vi "Unsigned Unsafe Subtract.vi"(1 "B":T1={"Array Num"=[1, 2, 3], "Decimal Index"=0, "stop"=FALSE}, 2 "A":T1={"Array Num"=[1, 2, 3], "Decimal Index"=0, "stop"=FALSE}) -> (0 "A-B":T1={"Array Num"=[1, 2, 3], "Decimal Index"=0, "stop"=FALSE})   [LabVIEW 2025]
uses:
  Number.ctl
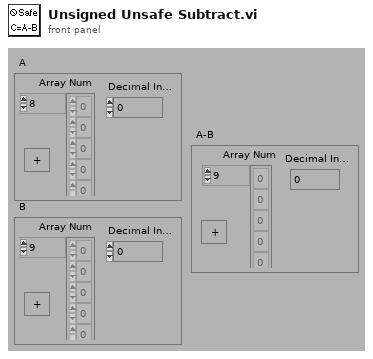
[diagram p1: front panel]
types:
  T1 = typedef "Number.ctl" = cluster{"Array Num":i8[], "Decimal Index":i32, "stop":bool}
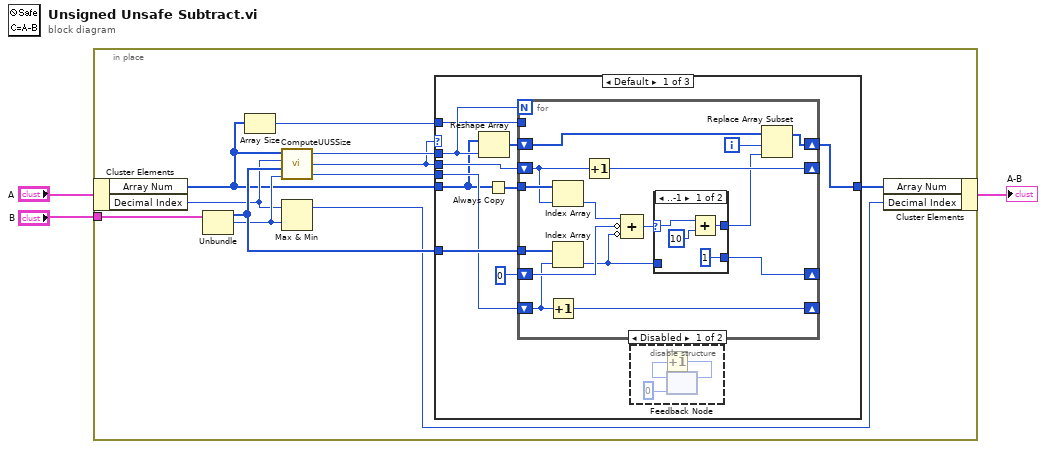
[diagram p0: block diagram]
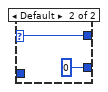
[diagram p3: hidden frame]
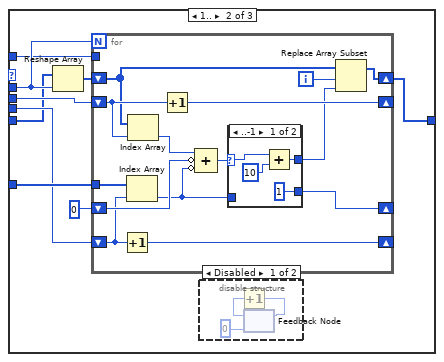
[diagram p4: hidden frame]
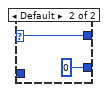
[diagram p6: hidden frame]
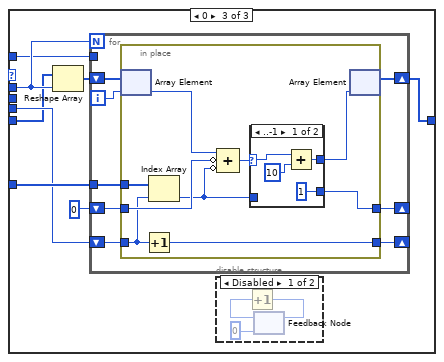
[diagram p7: hidden frame]
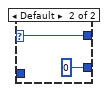
[diagram p9: hidden frame]
diagram:
  n1 = in-place {
    in-place-border: "B" -> [w14]
    n2 = in-place-cluster #1("A") -> ("Array Num"=w6:i8[], "Decimal Index"=w10:i32)
    n3 = Unbundle(w14) -> ("Array Num"=w13:i8[], "Decimal Index"=w12:i32)  [unwired: 1 out]
    n4 = Array Size(array=w6) -> (size(s)=w5:i32)
    n5 = call "ComputeUUSSize.vi"("B Array Position"=w12, "BArray"=w13, "A Array Position"=w10, "A Array Num"=w6) -> ("B Index"=w11:i32, "A Index"=w4:i32, "Loop Count"=w8:i32)
    n6 = Max & Min(x=w10, y=w12) -> (max(x,y)=w9:i32)  [unwired: 1 out]
    n7 = case shown="Default" w4 {
      tunnel: w13 -> [w23 w56 w87]
      tunnel: w4 -> [w22 w55 _]
      tunnel: w11 -> [w21 w54 w86]
      tunnel: w8 -> [w19 w53 w85]
      tunnel: [w17 w51 w83] -> w7
      tunnel: w6 -> [w16 w50 w81]
      tunnel: w5 -> [w15 w49 w82]
      frame Default {
        n8 = Reshape Array(w16, w19) -> (w18:i8[])
        n9 = Always Copy(1:w16) -> (0:w20:i8[])
        n10 = for {
          N: w19 -> [_]
          tunnel: w23 -> [w42]
          shift-right: [w41] -> _
          shift-left: i8 0 -> [w35]
          tunnel: w20 -> [w40]
          shift-right: [w37] -> _
          shift-left: w22 -> [w39]
          shift-right: [w38] -> _
          shift-left: w21 -> [w32]
          shift-right: [w30] -> w17
          shift-left: w18 -> [w31]
          tunnel: w15 -> [_]
          i -> [w29]
          n11 = Increment(x=w32) -> (x+1=w38:i32)
          n12 = Index Array(array=w40, index=w39) -> (element=w36:i8)
          n13 = Index Array(array=w42, index=w32) -> (element=w34:i8)
          n14 = Increment(x=w39) -> (x+1=w37:i32)
          n15 = Compound Arithmetic op=ADD(w36, invert w35, invert w34) -> (w33:i8)
          n16 = case shown="..-1" w33 {
            selector: w33 -> [w43 w47]
            tunnel: w34 -> [_ _]
            tunnel: [i8 1 i8 0] -> w41
            tunnel: [w44 w47] -> w28
            frame ..-1 {
              n17 = Add(x=w43, y=i8 10) -> (x+y=w44:i8)
            }
            frame Default {
            }
          }
          n18 = Replace Array Subset(array=w31, new element=w28, index=w29) -> (w30:i8[])
        }
        n19 = disable-structure shown="Disabled" {
          frame Disabled {
            n20 = feedback #2(0) -> (w26:i32)
            n21 = Increment(x=w26) -> (x+1=w27:i32)
            n22 = feedback-in #2(w27) -> ()
          }
          frame Enabled {
          }
        }
      }
      frame 1.. {
        n23 = Reshape Array(w50, w53) -> (w52:i8[])
        n24 = for {
          N: w53 -> [_]
          tunnel: w56 -> [w74]
          shift-right: [w73] -> _
          shift-left: i8 0 -> [w68]
          shift-right: [w70] -> _
          shift-left: w55 -> [w72]
          shift-right: [w71] -> _
          shift-left: w54 -> [w65]
          shift-right: [w64] -> w51
          shift-left: w52 -> [w61]
          tunnel: w49 -> [_]
          i -> [w63]
          n25 = Increment(x=w65) -> (x+1=w71:i32)
          n26 = Index Array(array=w74, index=w65) -> (element=w67:i8)
          n27 = Index Array(array=w61, index=w72) -> (element=w69:i8)
          n28 = Increment(x=w72) -> (x+1=w70:i32)
          n29 = Compound Arithmetic op=ADD(w69, invert w68, invert w67) -> (w66:i8)
          n30 = case shown="..-1" w66 {
            selector: w66 -> [w75 w79]
            tunnel: w67 -> [_ _]
            tunnel: [i8 1 i8 0] -> w73
            tunnel: [w76 w79] -> w62
            frame ..-1 {
              n31 = Add(x=w75, y=i8 10) -> (x+y=w76:i8)
            }
            frame Default {
            }
          }
          n32 = Replace Array Subset(array=w61, new element=w62, index=w63) -> (w64:i8[])
        }
        n33 = disable-structure shown="Disabled" {
          frame Disabled {
            n34 = feedback #3(0) -> (w58:i32)
            n35 = Increment(x=w58) -> (x+1=w59:i32)
            n36 = feedback-in #3(w59) -> ()
          }
          frame Enabled {
          }
        }
      }
      frame 0 {
        n37 = Reshape Array(w81, w85) -> (w84:i8[])
        n38 = for {
          N: w85 -> [_]
          tunnel: w87 -> [w99]
          shift-right: [w98] -> _
          shift-left: i8 0 -> [w96]
          shift-right: [w97] -> _
          shift-left: w86 -> [w95]
          shift-right: [w92] -> w83
          shift-left: w84 -> [w94]
          tunnel: w82 -> [_]
          i -> [w93]
          n39 = in-place {
            in-place-border: w99 -> [w108]
            in-place-border: [w107] -> w98
            in-place-border: [w106] -> w97
            in-place-border: w96 -> [w105]
            in-place-border: w95 -> [w102]
            n40 = in-place-array #4(w94, w93) -> (w100:i8)
            n41 = Increment(x=w102) -> (x+1=w106:i32)
            n42 = Index Array(array=w108, index=w102) -> (element=w104:i8)
            n43 = Compound Arithmetic op=ADD(w100, invert w105, invert w104) -> (w103:i8)
            n44 = case shown="..-1" w103 {
              selector: w103 -> [w109 w113]
              tunnel: w104 -> [_ _]
              tunnel: [i8 1 i8 0] -> w107
              tunnel: [w110 w113] -> w101
              frame ..-1 {
                n45 = Add(x=w109, y=i8 10) -> (x+y=w110:i8)
              }
              frame Default {
              }
            }
            n46 = in-place-array #4(w101) -> (w92:i8[])  [unwired: 1 out]
          }
        }
        n47 = disable-structure shown="Disabled" {
          frame Disabled {
            n48 = feedback #5(0) -> (w89:i32)
            n49 = Increment(x=w89) -> (x+1=w90:i32)
            n50 = feedback-in #5(w90) -> ()
          }
          frame Enabled {
          }
        }
      }
    }
    n51 = in-place-cluster #1("Array Num"=w7, "Decimal Index"=w9) -> (→"A-B":T1)
  }
